vi "水样测试.vi"(11 "数据标记表":string(combo)="N") -> ()   [LabVIEW 2016, in "斯坦道多参数.lvlib"]
panel:
  out "运行状态":u16(ring) items=["空闲", "水样测试", "标样核查"]
  out "多参数运行日志":string
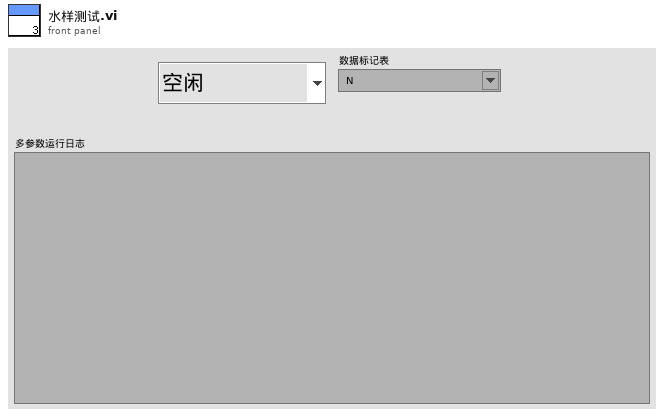
[diagram p1: front panel]
types:
  T1 = cluster{"水温":bool, "pH":bool, "DO":bool, "DOper":bool, "电导率":bool, "ORP":bool, "浊度":bool, "叶绿素a":bool, "藻密度":bool}
  T2 = cluster{"水样数据时间":timestamp, "检测值":cluster{"水温":dbl, "pH":dbl, "DO":dbl, "DOper":dbl, "电导率":dbl, "ORP":dbl, "浊度":dbl, "叶绿素a":dbl, "藻密度":dbl}}
  T3 = cluster{"水样数据时间":timestamp, "水样实测值":sgl, "单位":string, "水样数据标识":string, "信号值":sgl, "标样参考值":sgl, "因子编码":string, "探头温度":sgl}
  T4 = cluster{"ph":bool, "DO":bool, "Cond":bool, "Turb":bool, "叶绿素a":bool, "藻密度":bool, "ORP":bool}
  T5 = cluster{"CH":u16, "监测值":dbl, "温度偏移修正值":sgl, "信号值":sgl}
  T6 = cluster{"温度测量值":sgl, "测量值":sgl, "温度偏移修正值":sgl, "信号值":sgl}
  T7 = cluster{"温度测量值":sgl, "DO%":sgl, "DOmg/L":sgl, "温度偏移修正值":sgl}
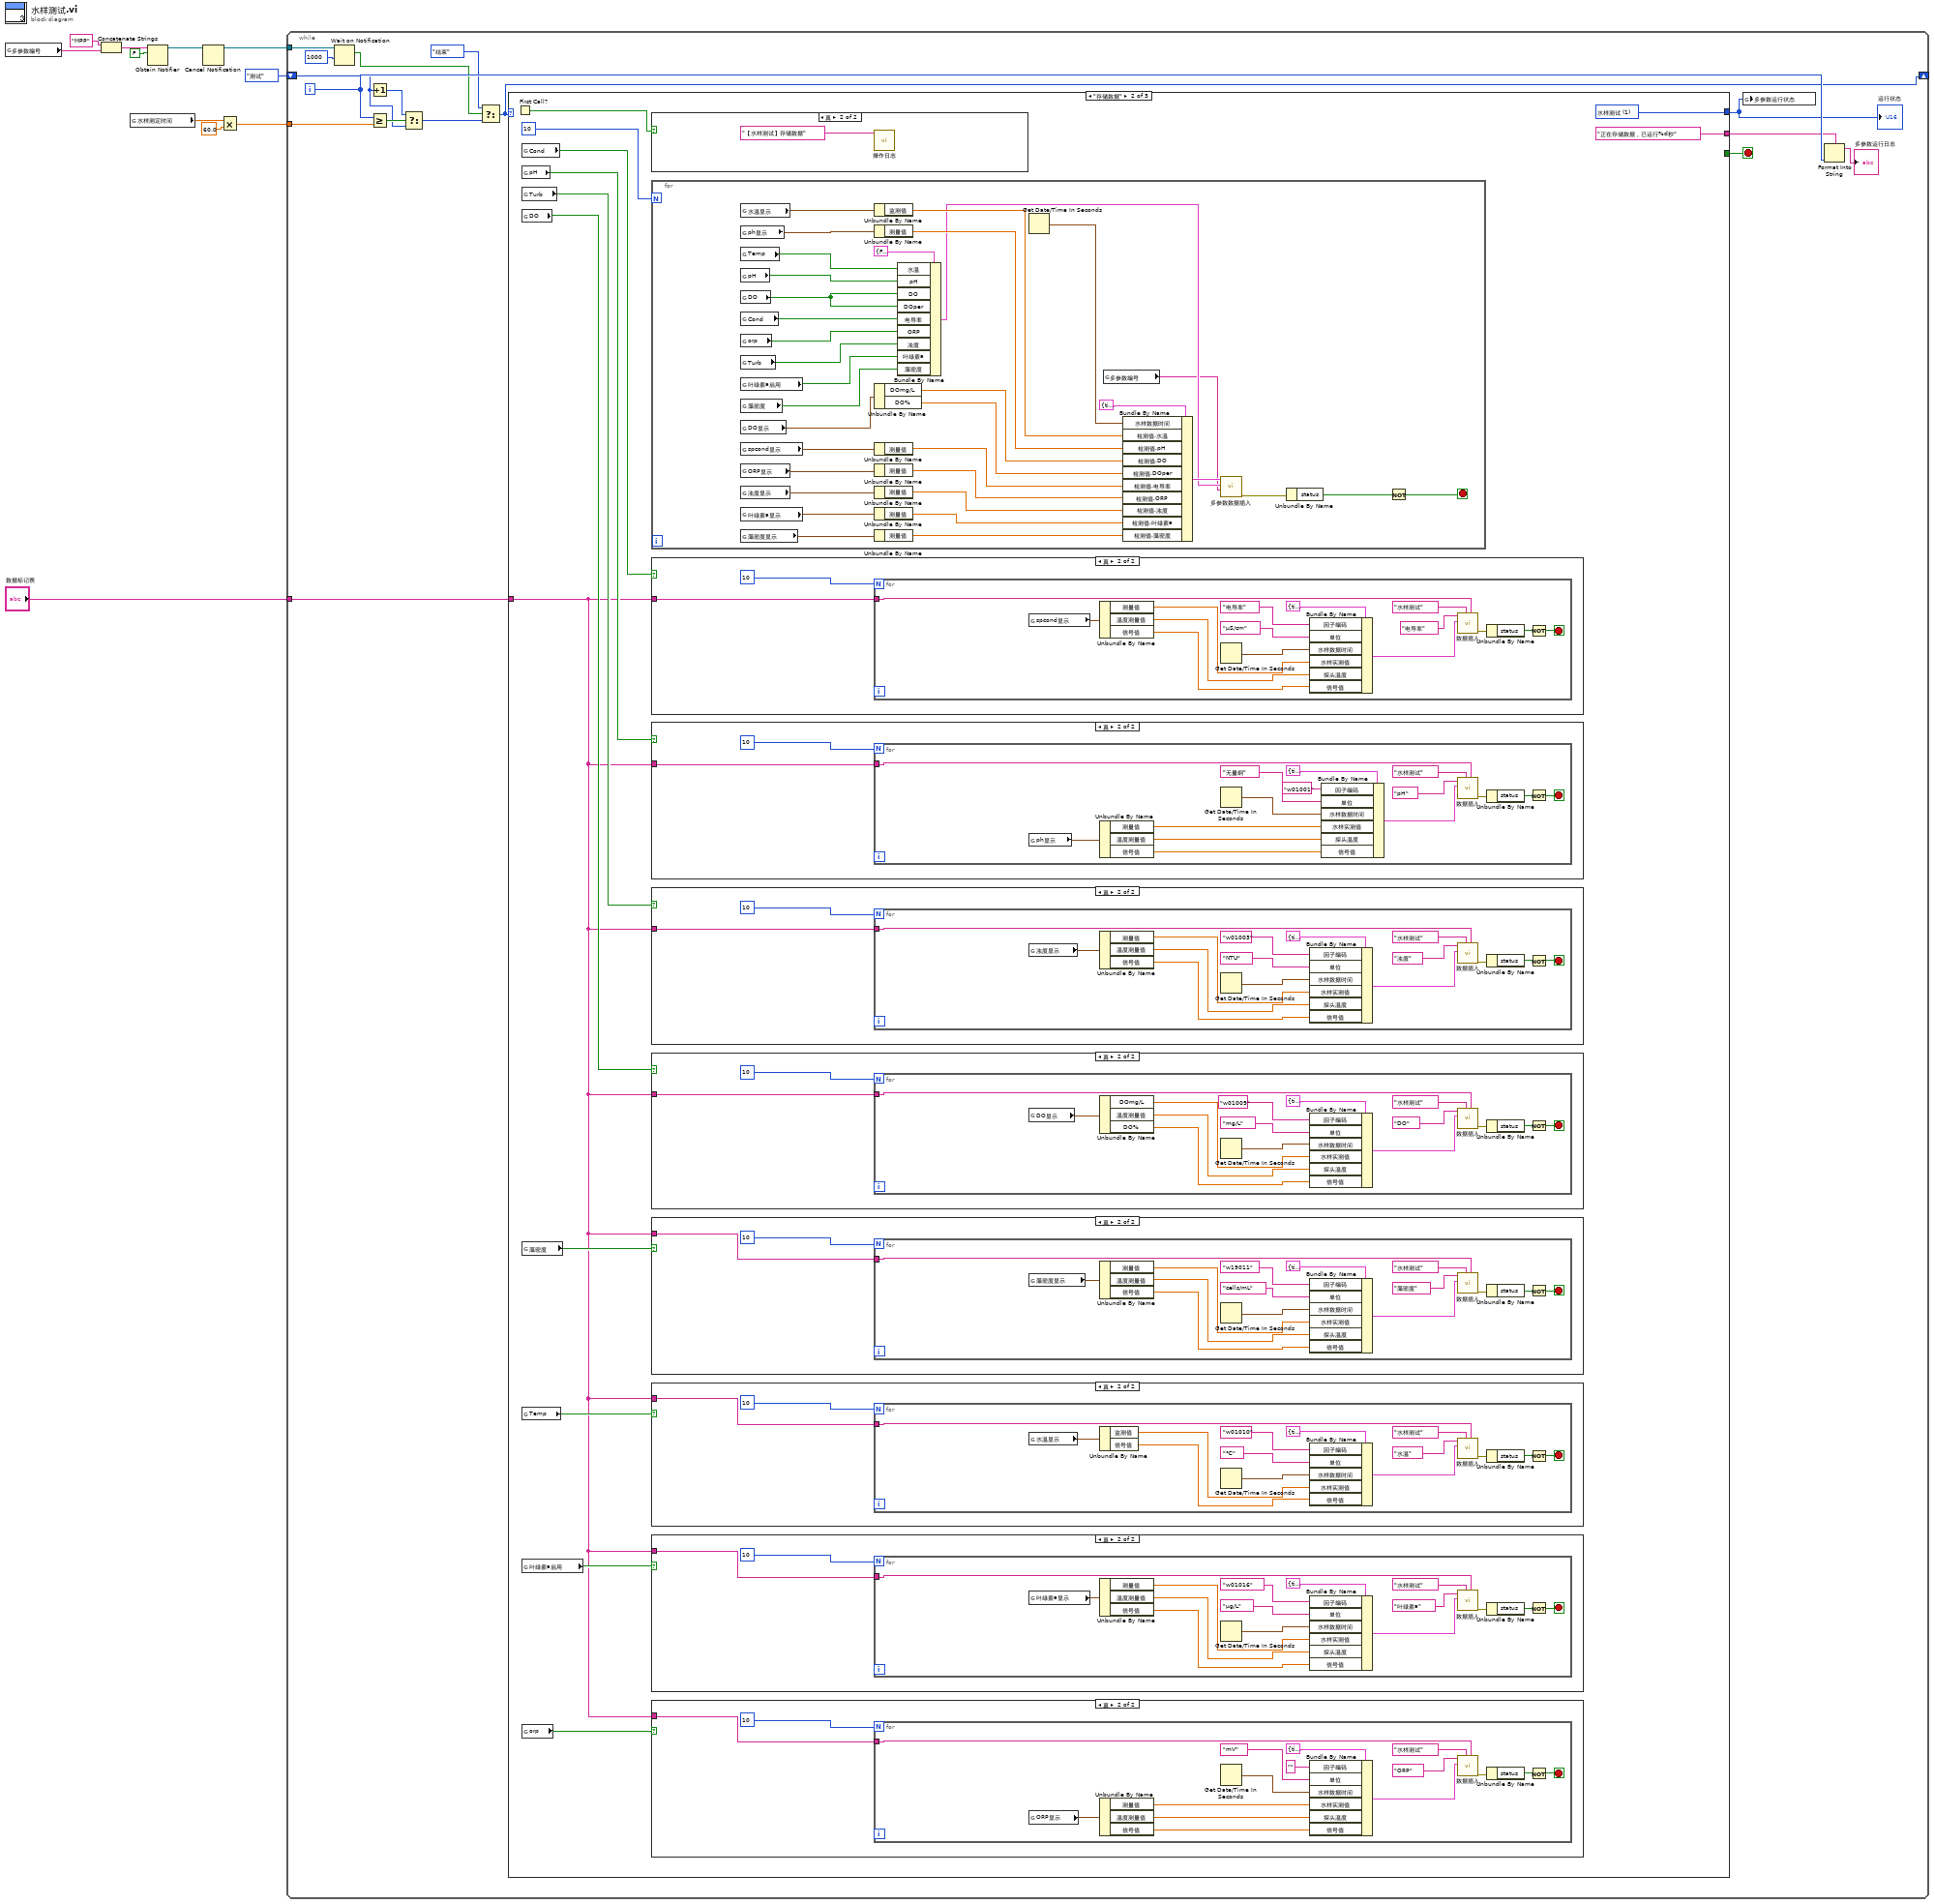
[diagram p0: block diagram]
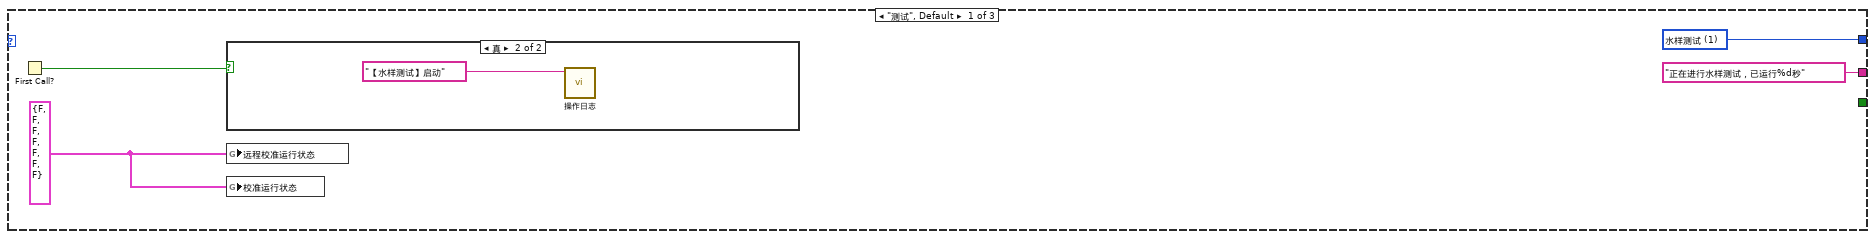
[diagram p2: hidden frame]
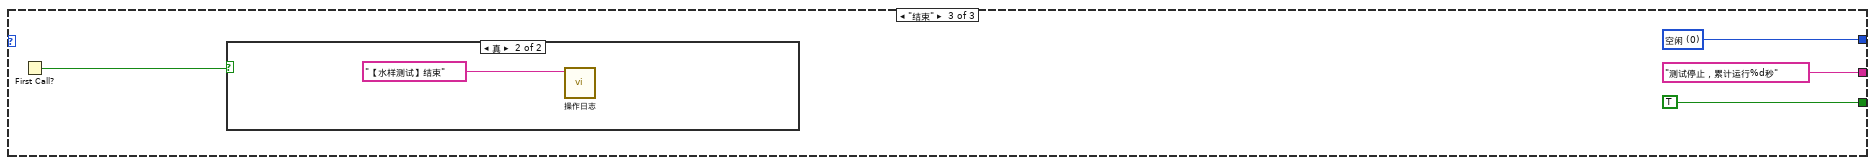
[diagram p13: hidden frame]
diagram:
  n1 = global read "多参数全局变量.vi" "多参数编号"() -> (w2:string)
  n2 = Concatenate Strings("MPP" ("名称（未命名）"), w2) -> (w3:string)
  n3 = global read "断电保存变量.vi" "水样测定时间"() -> (w1:dbl)
  n4 = Obtain Notifier(name (unnamed)=w3, notification data type=FALSE) -> (notifier out=w6:refnum<notifier>)  [unwired: 2 in, 2 out]
  n5 = Cancel Notification(0:w6) -> (8:w5:refnum<notifier>)  [unwired: 1 in, 2 out]
  n6 = Multiply(x=w1, y=60.0) -> (x*y=w10:dbl)
  n7 = while {
    tunnel: w10 -> [w27]
    shift-right: [w14] -> _
    shift-left: enum16{"测试", "存储数据", "结束"}."测试" ("枚举") -> [w21]
    tunnel: w5 -> [w19]
    tunnel: "数据标记表" -> [w13]
    i -> [w25]
    stop <- w26 stop-if-true
    n8 = Wait on Notification(notifier=w19, timeout in ms (-1)=1000 ("超时毫秒(-1)")) -> (notification=w17:bool)  [unwired: 2 in, 3 out]
    n9 = Increment(x=w21) -> (x+1=w20:enum16{"测试", "存储数据", "结束"})
    n10 = Greater Or Equal?(x=w25, y=w27) -> (x >= y?=w22:bool)
    n11 = Select(t=w20, s=w22, f=w21) -> (s? t:f=w15:enum16{"测试", "存储数据", "结束"})
    n12 = Select(t=enum16{"测试", "存储数据", "结束"}."结束" ("枚举"), s=w17, f=w15) -> (s? t:f=w14:enum16{"测试", "存储数据", "结束"})
    n13 = case shown="\"存储数据\"" w14 {
      tunnel: [_ _ TRUE] -> w26
      tunnel: ["正在进行水样测试，已运行%d秒" ("格式字符串") "正在存储数据，已运行%d秒" ("格式字符串") "测试停止，累计运行%d秒" ("格式字符串")] -> w24
      tunnel: [w30 w38 w217] -> w12
      tunnel: w13 -> [_ w35 _]
      frame "测试", Default {
        w28 = T4 {"ph"=FALSE, "DO"=FALSE, "Cond"=FALSE, "Turb"=FALSE, "叶绿素a"=FALSE, "藻密度"=FALSE, "ORP"=FALSE} ("校准运行状态")
        w30 = u16 1 items=["空闲", "水样测试", "标样核查"] ("多参数运行状态")
        n14 = First Call?() -> (First Call?: T/F=w29:bool)
        n15 = case shown="真" w29 {
          frame False {
          }
          frame True {
            n16 = call "操作日志.vi"("日志信息"="【水样测试】启动") -> ()  [unwired: 10 in, 1 out]
          }
        }
        n17 = global write "多参数全局变量.vi" "远程校准运行状态"(w28) -> ()
        n18 = global write "多参数全局变量.vi" "校准运行状态"(w28) -> ()
      }
      frame "存储数据" {
        w38 = u16 1 items=["空闲", "水样测试", "标样核查"] ("多参数运行状态")
        n19 = First Call?() -> (First Call?: T/F=w36:bool)
        n20 = global read "断电保存变量.vi" "Cond"() -> (w43:bool)
        n21 = global read "断电保存变量.vi" "pH"() -> (w41:bool)
        n22 = global read "断电保存变量.vi" "Turb"() -> (w44:bool)
        n23 = global read "断电保存变量.vi" "DO"() -> (w42:bool)
        n24 = global read "断电保存变量.vi" "藻密度"() -> (w37:bool)
        n25 = global read "断电保存变量.vi" "Temp"() -> (w40:bool)
        n26 = global read "断电保存变量.vi" "叶绿素a启用"() -> (w45:bool)
        n27 = global read "断电保存变量.vi" "orp"() -> (w34:bool)
        n28 = case shown="真" w36 {
          frame False {
          }
          frame True {
            n29 = call "操作日志.vi"("日志信息"="【水样测试】存储数据") -> ()  [unwired: 10 in, 1 out]
          }
        }
        n30 = for {
          N: 10 -> [_]
          stop <- w47 stop-if-true
          n31 = global read "多参数全局变量.vi" "水温显示"() -> (w76:T5)
          n32 = global read "多参数全局变量.vi" "ph显示"() -> (w74:T6)
          n33 = global read "断电保存变量.vi" "Temp"() -> (w54:bool)
          n34 = global read "断电保存变量.vi" "pH"() -> (w58:bool)
          n35 = global read "断电保存变量.vi" "DO"() -> (w50:bool)
          n36 = global read "断电保存变量.vi" "Cond"() -> (w57:bool)
          n37 = global read "断电保存变量.vi" "orp"() -> (w53:bool)
          n38 = global read "断电保存变量.vi" "Turb"() -> (w56:bool)
          n39 = global read "断电保存变量.vi" "叶绿素a启用"() -> (w52:bool)
          n40 = global read "断电保存变量.vi" "藻密度"() -> (w55:bool)
          n41 = global read "多参数全局变量.vi" "DO显示"() -> (w72:T7)
          n42 = global read "多参数全局变量.vi" "spcond显示"() -> (w69:T6)
          n43 = global read "多参数全局变量.vi" "ORP显示"() -> (w67:T6)
          n44 = global read "多参数全局变量.vi" "浊度显示"() -> (w65:T6)
          n45 = global read "多参数全局变量.vi" "叶绿素a显示"() -> (w61:T6)
          n46 = global read "多参数全局变量.vi" "藻密度显示"() -> (w63:T6)
          n47 = Unbundle By Name(w76) -> ("监测值"=w75:dbl)
          n48 = Unbundle By Name(w74) -> ("测量值"=w73:sgl)
          n49 = Unbundle By Name(w72) -> ("DOmg/L"=w71:sgl, "DO%"=w70:sgl)
          n50 = Unbundle By Name(w69) -> ("测量值"=w68:sgl)
          n51 = Unbundle By Name(w67) -> ("测量值"=w66:sgl)
          n52 = Unbundle By Name(w65) -> ("测量值"=w64:sgl)
          n53 = Unbundle By Name(w61) -> ("测量值"=w60:sgl)
          n54 = Unbundle By Name(w63) -> ("测量值"=w62:sgl)
          n55 = Bundle By Name(cluster=T1 {"水温"=FALSE, "pH"=FALSE, "DO"=FALSE, "DOper"=FALSE, "电导率"=FALSE, "ORP"=FALSE, "浊度"=FALSE, "叶绿素a"=FALSE, "藻密度"=FALSE} ("columns enable"), "水温"=w54, "pH"=w58, "DO"=w50, "DOper"=w50, "电导率"=w57, "ORP"=w53, "浊度"=w56, "叶绿素a"=w52, "藻密度"=w55) -> (w51:T1)
          n56 = Get Date/Time In Seconds() -> (seconds since 1Jan1904=w77:timestamp)
          n57 = global read "多参数全局变量.vi" "多参数编号"() -> (w46:string)
          n58 = Bundle By Name(cluster=T2 {"水样数据时间"=timestamp(0 s since 1904-01-01), "检测值"={"水温"=0.0, "pH"=0.0, "DO"=0.0, "DOper"=0.0, "电导率"=0.0, "ORP"=0.0, "浊度"=0.0, "叶绿素a"=0.0, "藻密度"=0.0}} ("data in"), "水样数据时间"=w77, "检测值.水温"=w75, "检测值.pH"=w73, "检测值.DO"=w71, "检测值.DOper"=w70, "检测值.电导率"=w68, "检测值.ORP"=w66, "检测值.浊度"=w64, "检测值.叶绿素a"=w60, "检测值.藻密度"=w62) -> (w78:T2)
          n59 = call "多参数数据插入.vi"("编号"=w46, "columns enable"=w51, "data in"=w78) -> ("error out"=w49:errorcluster)  [unwired: 8 in]
          n60 = Unbundle By Name(w49) -> ("status"=w48:bool)
          n61 = Not(x=w48) -> (.not. x?=w47:bool)
        }
        n62 = case shown="真" w43 {
          tunnel: w35 -> [_ w150]
          frame False {
          }
          frame True {
            n63 = for {
              N: 10 -> [_]
              tunnel: w150 -> [w160]
              stop <- w154 stop-if-true
              n64 = global read "多参数全局变量.vi" "spcond显示"() -> (w159:T6)
              n65 = Unbundle By Name(w159) -> ("测量值"=w158:sgl, "温度测量值"=w157:sgl, "信号值"=w151:sgl)
              n66 = Get Date/Time In Seconds() -> (seconds since 1Jan1904=w163:timestamp)
              n67 = Bundle By Name(cluster=T3 {"水样数据时间"=timestamp(0 s since 1904-01-01), "水样实测值"=0.0, "单位"="", "水样数据标识"="N", "信号值"=0.0, "标样参考值"=0.0, "因子编码"="", "探头温度"=0.0} ("data in"), "因子编码"="电导率", "单位"="μS/cm", "水样数据时间"=w163, "水样实测值"=w158, "探头温度"=w157, "信号值"=w151) -> (w164:T3)
              n68 = call "数据插入.vi"("数据类型"=w160, "测量模式"="水样测试", "data in"=w164, "table输入"="电导率") -> ("error out"=w156:errorcluster)  [unwired: 7 in]
              n69 = Unbundle By Name(w156) -> ("status"=w155:bool)
              n70 = Not(x=w155) -> (.not. x?=w154:bool)
            }
          }
        }
        n71 = case shown="真" w41 {
          tunnel: w35 -> [_ w184]
          frame False {
          }
          frame True {
            n72 = for {
              N: 10 -> [_]
              tunnel: w184 -> [w193]
              stop <- w187 stop-if-true
              n73 = global read "多参数全局变量.vi" "ph显示"() -> (w192:T6)
              n74 = Unbundle By Name(w192) -> ("测量值"=w191:sgl, "温度测量值"=w190:sgl, "信号值"=w185:sgl)
              n75 = Get Date/Time In Seconds() -> (seconds since 1Jan1904=w197:timestamp)
              n76 = Bundle By Name(cluster=T3 {"水样数据时间"=timestamp(0 s since 1904-01-01), "水样实测值"=0.0, "单位"="", "水样数据标识"="N", "信号值"=0.0, "标样参考值"=0.0, "因子编码"="", "探头温度"=0.0} ("data in"), "因子编码"="w01001", "单位"="无量纲", "水样数据时间"=w197, "水样实测值"=w191, "探头温度"=w190, "信号值"=w185) -> (w198:T3)
              n77 = call "数据插入.vi"("数据类型"=w193, "测量模式"="水样测试", "data in"=w198, "table输入"="pH") -> ("error out"=w189:errorcluster)  [unwired: 7 in]
              n78 = Unbundle By Name(w189) -> ("status"=w188:bool)
              n79 = Not(x=w188) -> (.not. x?=w187:bool)
            }
          }
        }
        n80 = case shown="真" w44 {
          tunnel: w35 -> [_ w133]
          frame False {
          }
          frame True {
            n81 = for {
              N: 10 -> [_]
              tunnel: w133 -> [w142]
              stop <- w136 stop-if-true
              n82 = global read "多参数全局变量.vi" "浊度显示"() -> (w141:T6)
              n83 = Unbundle By Name(w141) -> ("测量值"=w140:sgl, "温度测量值"=w139:sgl, "信号值"=w134:sgl)
              n84 = Get Date/Time In Seconds() -> (seconds since 1Jan1904=w147:timestamp)
              n85 = Bundle By Name(cluster=T3 {"水样数据时间"=timestamp(0 s since 1904-01-01), "水样实测值"=0.0, "单位"="", "水样数据标识"="N", "信号值"=0.0, "标样参考值"=0.0, "因子编码"="", "探头温度"=0.0} ("data in"), "因子编码"="w01003", "单位"="NTU", "水样数据时间"=w147, "水样实测值"=w140, "探头温度"=w139, "信号值"=w134) -> (w146:T3)
              n86 = call "数据插入.vi"("数据类型"=w142, "测量模式"="水样测试", "data in"=w146, "table输入"="浊度") -> ("error out"=w138:errorcluster)  [unwired: 7 in]
              n87 = Unbundle By Name(w138) -> ("status"=w137:bool)
              n88 = Not(x=w137) -> (.not. x?=w136:bool)
            }
          }
        }
        n89 = case shown="真" w42 {
          tunnel: w35 -> [_ w167]
          frame False {
          }
          frame True {
            n90 = for {
              N: 10 -> [_]
              tunnel: w167 -> [w176]
              stop <- w170 stop-if-true
              n91 = global read "多参数全局变量.vi" "DO显示"() -> (w175:T7)
              n92 = Unbundle By Name(w175) -> ("DOmg/L"=w174:sgl, "温度测量值"=w173:sgl, "DO%"=w168:sgl)
              n93 = Get Date/Time In Seconds() -> (seconds since 1Jan1904=w181:timestamp)
              n94 = Bundle By Name(cluster=T3 {"水样数据时间"=timestamp(0 s since 1904-01-01), "水样实测值"=0.0, "单位"="", "水样数据标识"="N", "信号值"=0.0, "标样参考值"=0.0, "因子编码"="", "探头温度"=0.0} ("data in"), "因子编码"="w01009", "单位"="mg/L", "水样数据时间"=w181, "水样实测值"=w174, "探头温度"=w173, "信号值"=w168) -> (w180:T3)
              n95 = call "数据插入.vi"("数据类型"=w176, "测量模式"="水样测试", "data in"=w180, "table输入"="DO") -> ("error out"=w172:errorcluster)  [unwired: 7 in]
              n96 = Unbundle By Name(w172) -> ("status"=w171:bool)
              n97 = Not(x=w171) -> (.not. x?=w170:bool)
            }
          }
        }
        n98 = case shown="真" w37 {
          tunnel: w35 -> [_ w99]
          frame False {
          }
          frame True {
            n99 = for {
              N: 10 -> [_]
              tunnel: w99 -> [w107]
              stop <- w103 stop-if-true
              n100 = global read "多参数全局变量.vi" "藻密度显示"() -> (w106:T6)
              n101 = Unbundle By Name(w106) -> ("测量值"=w112:sgl, "温度测量值"=w110:sgl, "信号值"=w100:sgl)
              n102 = Get Date/Time In Seconds() -> (seconds since 1Jan1904=w113:timestamp)
              n103 = Bundle By Name(cluster=T3 {"水样数据时间"=timestamp(0 s since 1904-01-01), "水样实测值"=0.0, "单位"="", "水样数据标识"="N", "信号值"=0.0, "标样参考值"=0.0, "因子编码"="", "探头温度"=0.0} ("data in"), "因子编码"="w19011", "单位"="cells/mL", "水样数据时间"=w113, "水样实测值"=w112, "探头温度"=w110, "信号值"=w100) -> (w101:T3)
              n104 = call "数据插入.vi"("数据类型"=w107, "测量模式"="水样测试", "data in"=w101, "table输入"="藻密度") -> ("error out"=w105:errorcluster)  [unwired: 7 in]
              n105 = Unbundle By Name(w105) -> ("status"=w104:bool)
              n106 = Not(x=w104) -> (.not. x?=w103:bool)
            }
          }
        }
        n107 = case shown="真" w40 {
          tunnel: w35 -> [_ w201]
          frame False {
          }
          frame True {
            n108 = for {
              N: 10 -> [_]
              tunnel: w201 -> [w209]
              stop <- w204 stop-if-true
              n109 = global read "多参数全局变量.vi" "水温显示"() -> (w208:T5)
              n110 = Unbundle By Name(w208) -> ("监测值"=w207:dbl, "信号值"=w202:sgl)
              n111 = Get Date/Time In Seconds() -> (seconds since 1Jan1904=w214:timestamp)
              n112 = Bundle By Name(cluster=T3 {"水样数据时间"=timestamp(0 s since 1904-01-01), "水样实测值"=0.0, "单位"="", "水样数据标识"="N", "信号值"=0.0, "标样参考值"=0.0, "因子编码"="", "探头温度"=0.0} ("data in"), "因子编码"="w01010", "单位"="℃", "水样数据时间"=w214, "水样实测值"=w207, "信号值"=w202) -> (w213:T3)
              n113 = call "数据插入.vi"("数据类型"=w209, "测量模式"="水样测试", "data in"=w213, "table输入"="水温") -> ("error out"=w206:errorcluster)  [unwired: 7 in]
              n114 = Unbundle By Name(w206) -> ("status"=w205:bool)
              n115 = Not(x=w205) -> (.not. x?=w204:bool)
            }
          }
        }
        n116 = case shown="真" w45 {
          tunnel: w35 -> [_ w116]
          frame False {
          }
          frame True {
            n117 = for {
              N: 10 -> [_]
              tunnel: w116 -> [w124]
              stop <- w120 stop-if-true
              n118 = global read "多参数全局变量.vi" "叶绿素a显示"() -> (w123:T6)
              n119 = Unbundle By Name(w123) -> ("测量值"=w129:sgl, "温度测量值"=w128:sgl, "信号值"=w117:sgl)
              n120 = Get Date/Time In Seconds() -> (seconds since 1Jan1904=w130:timestamp)
              n121 = Bundle By Name(cluster=T3 {"水样数据时间"=timestamp(0 s since 1904-01-01), "水样实测值"=0.0, "单位"="", "水样数据标识"="N", "信号值"=0.0, "标样参考值"=0.0, "因子编码"="", "探头温度"=0.0} ("data in"), "因子编码"="w01016", "单位"="μg/L", "水样数据时间"=w130, "水样实测值"=w129, "探头温度"=w128, "信号值"=w117) -> (w126:T3)
              n122 = call "数据插入.vi"("数据类型"=w124, "测量模式"="水样测试", "data in"=w126, "table输入"="叶绿素a") -> ("error out"=w122:errorcluster)  [unwired: 7 in]
              n123 = Unbundle By Name(w122) -> ("status"=w121:bool)
              n124 = Not(x=w121) -> (.not. x?=w120:bool)
            }
          }
        }
        n125 = case shown="真" w34 {
          tunnel: w35 -> [_ w81]
          frame False {
          }
          frame True {
            n126 = for {
              N: 10 -> [_]
              tunnel: w81 -> [w89]
              stop <- w85 stop-if-true
              n127 = global read "多参数全局变量.vi" "ORP显示"() -> (w88:T6)
              n128 = Unbundle By Name(w88) -> ("测量值"=w94:sgl, "温度测量值"=w92:sgl, "信号值"=w82:sgl)
              n129 = Get Date/Time In Seconds() -> (seconds since 1Jan1904=w95:timestamp)
              n130 = Bundle By Name(cluster=T3 {"水样数据时间"=timestamp(0 s since 1904-01-01), "水样实测值"=0.0, "单位"="", "水样数据标识"="N", "信号值"=0.0, "标样参考值"=0.0, "因子编码"="", "探头温度"=0.0} ("data in"), "因子编码"="", "单位"="mV", "水样数据时间"=w95, "水样实测值"=w94, "探头温度"=w92, "信号值"=w82) -> (w90:T3)
              n131 = call "数据插入.vi"("数据类型"=w89, "测量模式"="水样测试", "data in"=w90, "table输入"="ORP") -> ("error out"=w87:errorcluster)  [unwired: 7 in]
              n132 = Unbundle By Name(w87) -> ("status"=w86:bool)
              n133 = Not(x=w86) -> (.not. x?=w85:bool)
            }
          }
        }
      }
      frame "结束" {
        w217 = u16 0 items=["空闲", "水样测试", "标样核查"] ("多参数运行状态")
        n134 = First Call?() -> (First Call?: T/F=w216:bool)
        n135 = case shown="真" w216 {
          frame False {
          }
          frame True {
            n136 = call "操作日志.vi"("日志信息"="【水样测试】结束") -> ()  [unwired: 10 in, 1 out]
          }
        }
      }
    }
    "运行状态" <- w12
    n137 = global write "多参数全局变量.vi" "多参数运行状态"(w12) -> ()
    n138 = Format Into String(format string=w24, w25) -> (resulting string=→"多参数运行日志":string)  [unwired: 2 in, 1 out]
  }
